vi "Right Motor ENC.vi"(0 "SPI Config In":T1) -> (1 "SPI Config Out":T1, 2 "Motor Pos":fxp<+,51,11>)   [LabVIEW 2019]
uses:
  SPI/SPI Config.ctl
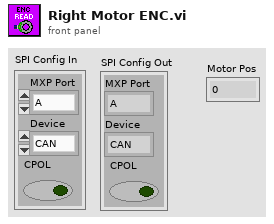
[diagram p1: front panel]
types:
  T1 = typedef "SPI Config.ctl" = cluster{"MXP Port":enum16{"A", "B"}, "Device":enum16{"CAN", "ENC", "IMU1", "IMU2"}, "CPOL":bool}
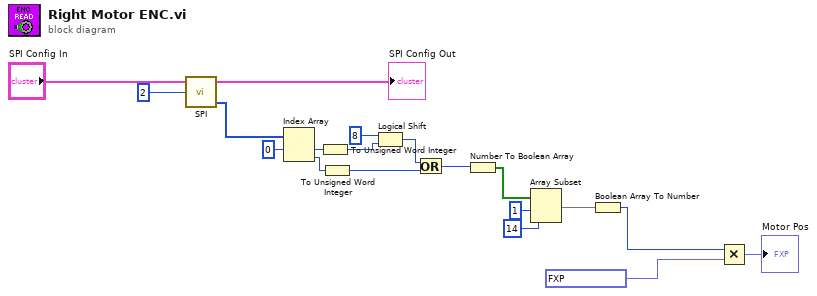
[diagram p0: block diagram]
diagram:
  n1 = call "SPI.vi"("Frames to Write"=u8 2, "SPI Config In"="SPI Config In") -> ("Data Read"=w15:u8[], "SPI Config Out"=→"SPI Config Out":T1)  [unwired: 1 in, 1 out]
  n2 = Index Array(array=w15, index #1=0 ("index")) -> (element #1=w14:u8, element #2=w13:u8)  [unwired: 1 in]
  n3 = To Unsigned Word Integer(number=w14) -> (unsigned 16bit integer=w11:u16)
  n4 = To Unsigned Word Integer(number=w13) -> (unsigned 16bit integer=w9:u16)
  n5 = Logical Shift(y=i16 8, x=w11) -> (x << y=w10:u16)
  n6 = Or(x=w10, y=w9) -> (x .or. y?=w8:u16)
  n7 = Number To Boolean Array(number=w8) -> (Boolean array=w7:bool[])
  n8 = Array Subset(array=w7, index=1, length=14) -> (w4:bool[])
  n9 = Boolean Array To Number(Boolean array=w4) -> (number=w2:u16)
  n10 = Multiply(x=w2, y=fxp<+,35,-5> 0.021973997429995507) -> (x*y=→"Motor Pos":fxp<+,51,11>)
